vi "StopSignal-StopFilteredSignalsInDefaultOrder.vi"(6 "filter signal":string[](array[string]), 8 "error in (no error)":errorcluster, 9 "interval time(ms)":u32, 10 "reason(\"\")":string, 11 "Reverse？":bool) -> (0 "error out":errorcluster)   [LabVIEW 2017, in "StopSignal.lvlib"]
uses:
  StopSignal.lvlib
  C/Program Files (x86)/National Instruments/LabVIEW 2019/user.lib/_OpenG.lib/array/array.llb/Filter 1D Array (String)__ogtk.vi
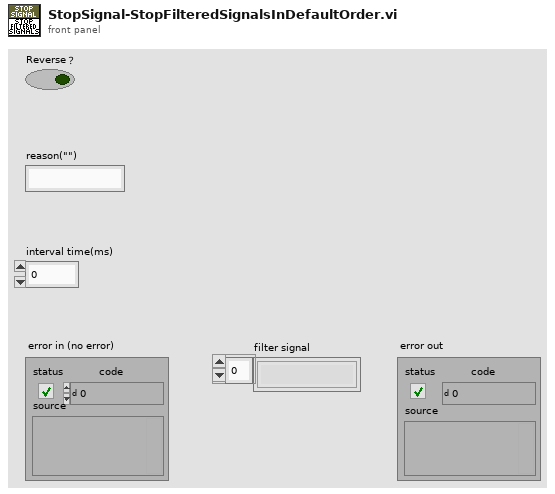
[diagram p1: front panel]
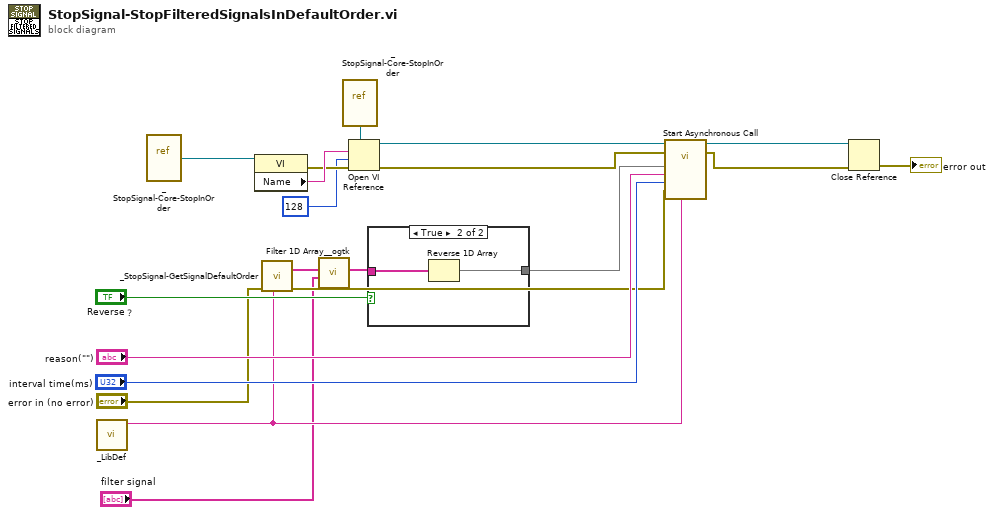
[diagram p0: block diagram]
diagram:
  n1 = call "_LibDef.vi"() -> ("LIBNAME"=w4:string)  [unwired: 11 in]
  n2 = vi-ref "_StopSignal-Core-StopInOrder.vi"() -> (w18:refnum<vi>)
  n3 = property class="VI"(reference=w18) -> (error out=w19:errorcluster, "Name"=w20:string)  [unwired: 1 in, 1 out]
  n4 = call "_StopSignal-GetSignalDefaultOrder.vi"("LIBNAME"=w4, "error in (no error)"="error in (no error)") -> ("error out"=w6:errorcluster, "SignalInArray"=w3:string[])  [unwired: 8 in]
  n5 = call-poly "Filter 1D Array__ogtk.vi"("items to filter"="filter signal", "array"=w3) -> ("filtered array"=w1:string[])  [unwired: 4 in, 1 out]
  n6 = vi-ref "_StopSignal-Core-StopInOrder.vi"() -> (w17:refnum<vi>)
  n7 = Open VI Reference(type specifier VI Refnum (for type only)=w17, vi path=w20, options=128, error in (no error)=w19) -> (vi reference=w16:refnum<vi>, error out=w15:errorcluster)  [unwired: 2 in]
  n8 = case shown="True" "Reverse？" {
    tunnel: w1 -> [w21 w23]
    tunnel: [w21 w22] -> w5
    frame False {
    }
    frame True {
      n9 = Reverse 1D Array(array=w23) -> (reversed array=w22:string[])
    }
  }
  n10 = call-by-ref "Start Asynchronous Call"(reference=w16, error in=w15, "LIBNAME"=w4, 8:"error in (no error)"=w6, "interval time(ms)"="interval time(ms)", "reason(\"\")"="reason(\"\")", "name(\"\")"=w5) -> (reference out=w13:refnum<vi>, error out=w14:errorcluster)  [unwired: 5 in, 2 out]
  n11 = Close Reference(reference=w13, error in (no error)=w14) -> (error out=→"error out":errorcluster)
